vi "LEDs.vi"(11 "Enum":T1(ring)) -> ()   [LabVIEW 2017]
uses:
  <vilib>/myRIO/Instrument Drivers/Onboard IO/DIO/typedefs/DIO Reference.ctl
  <vilib>/myRIO/Common/Instrument Driver Framework/Utilities/typedefs/myRIO Generic Hardware Reference.ctl
  <vilib>/myRIO/Common/Instrument Driver Framework/Utilities/typedefs/Hardware Version Enum.ctl
  <vilib>/myRIO/Common/Instrument Driver Framework/Utilities/typedefs/myRIO v1.0 Reference.ctl
  <vilib>/myRIO/Common/Instrument Driver Framework/Utilities/typedefs/Generic FPGA Reference.ctl
  <vilib>/myRIO/Common/Instrument Driver Framework/myRIO v1.0/DIO/typedefs/DIO Channels List.ctl
  <vilib>/myRIO/Common/Instrument Driver Framework/myRIO v1.0/DIO/typedefs/DIO Channels Enum.ctl
  <vilib>/userdefined/High Color/nirio_resource_hc.ctl
  <vilib>/myRIO/Common/Instrument Driver Framework/Utilities/vis/Is FPGA Ref Available.vi
  <vilib>/myRIO/Common/Instrument Driver Framework/myRIO v1.0/DIO/vis/myRIO v1.1 Open DIO.vi
  <vilib>/myRIO/Instrument Drivers/Onboard IO/DIO/vis/Write.vi
  <vilib>/myRIO/Common/Instrument Driver Framework/Utilities/vis/Validate Channels.vi
  <vilib>/myRIO/Common/Instrument Driver Framework/myRIO v1.0/DIO/vis/myRIO v1.0 Reserve DIO.vi
  <vilib>/myRIO/Common/Instrument Driver Framework/myRIO v1.0/Resource Manager/vis/myRIO v1.0 Reserve Channel List.vi
  <vilib>/myRIO/Common/Instrument Driver Framework/myRIO v1.0/DIO/vis/myRIO v1.0 Build MUX Configuration DIO.vi
  <vilib>/myRIO/Common/Instrument Driver Framework/myRIO v1.0/Resource Manager/vis/myRIO v1.0 Reserve Channel.vi
  <vilib>/myRIO/Common/Instrument Driver Framework/myRIO v1.0/Resource Manager/vis/myRIO v1.0 Unreserve Channel.vi
  <vilib>/myRIO/Common/Instrument Driver Framework/myRIO v1.0/Resource Manager/vis/myRIO v1.0 Create Configuration List.vi
  <vilib>/myRIO/Common/Instrument Driver Framework/myRIO v1.0/Resource Manager/vis/myRIO v1.0 Build Mutex Name.vi
  <vilib>/Utility/VariantDataType/GetNumericInfo.vi
  <vilib>/Utility/error.llb/Error Cluster From Error Code.vi
  <vilib>/myRIO/Common/Instrument Driver Framework/myRIO v1.0/myRIO v1.1 Open.vi
  <vilib>/myRIO/Common/Instrument Driver Framework/Utilities/vis/IO Manager.vi
  <vilib>/myRIO/Common/Instrument Driver Framework/Utilities/vis/Configuration Manager.vi
  <vilib>/myRIO/Common/Instrument Driver Framework/myRIO v1.0/Resource Manager/vis/myRIO v1.0 Configure IO.vi
  <vilib>/myRIO/Common/Instrument Driver Framework/myRIO v1.0/myRIO v1.0 Close.vi
  <vilib>/myRIO/Common/Instrument Driver Framework/myRIO v1.0/DIO/vis/myRIO v1.0 Write DIO.vi
  <vilib>/myRIO/Express VI/Onboard IO/DO/DO Express VI.xnode
  <vilib>/myRIO/Instrument Drivers/Onboard IO/DIO/vis/myRIO DIO Open.xnode
  <vilib>/myRIO/Instrument Drivers/Onboard IO/DIO/DIO.lvlib
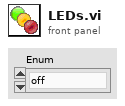
[diagram p1: front panel]
types:
  T1 = enum16{"off", "flash", "top", "middle", "bottom"}
  T2 = typedef "DIO.lvlib/DIO Reference.ctl" = cluster{"myRIO Reference":T3, "DIO Channels List":T7}
  T3 = typedef "myRIO Generic Hardware Reference.ctl" = cluster{"myRIO Model":T4, "myRIO Hardware Reference":T5}
  T4 = typedef "Hardware Version Enum.ctl" = enum16{"Unknown", "myRIO-1900", "myRIO-1950", "roboRIO", "NI ELVIS RIO CM"}
  T5 = typedef "myRIO v1.0 Reference.ctl" = cluster{"Generic FPGA Reference":T6, "Allow multiple opens":bool}
  T6 = typedef "Generic FPGA Reference.ctl" = refnum<k20>
  T7 = typedef "DIO Channels List.ctl" = T8[]
  T8 = typedef "DIO Channels Enum.ctl" = enum16{"Not Connected", "C/DIO0", "C/DIO1", "C/DIO2", "C/DIO3", "C/DIO4", "C/DIO5", "C/DIO6", "C/DIO7", "A/DIO0", "A/DIO1", "A/DIO2", "A/DIO3", "A/DIO4", "A/DIO5", "A/DIO6", "A/DIO7", "A/DIO8", "A/DIO9", "A/DIO10", "A/DIO11", "A/DIO12", "A/DIO13", "A/DIO14", "A/DIO15", "B/DIO0", "B/DIO1", "B/DIO2", "B/DIO3", "B/DIO4", "B/DIO5", "B/DIO6", "B/DIO7", "B/DIO8", "B/DIO9", "B/DIO10", "B/DIO11", "B/DIO12", "B/DIO13", "B/DIO14", "B/DIO15", "LED0", "LED1", "LED2", "LED3", "Button0", "DIO/DIO0", "DIO/DIO1", "DIO/DIO2", "DIO/DIO3", "DIO/DIO4", "DIO/DIO5", "DIO/DIO6", "DIO/DIO7", "DIO/DIO8", "DIO/DIO9", "SPI/CS0", "SPI/CS1", "SPI/CS2", "SPI/CS3", "LED RADIO (Green)", "LED RADIO (Red)", "LED COMM (Green)", "LED COMM (Red)", "LED MODE (Green)", "LED MODE (Red)"}
  T9 = typedef "nirio_resource_hc.ctl" = tag
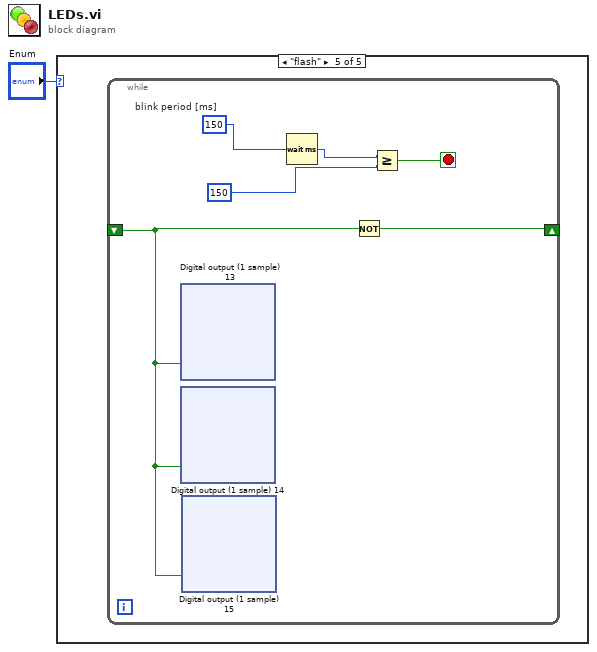
[diagram p0: block diagram]
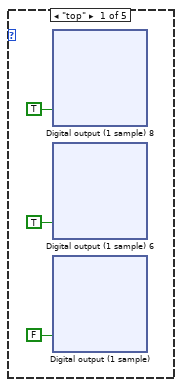
[diagram p2: hidden frame]
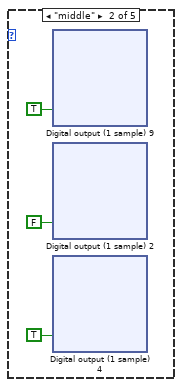
[diagram p3: hidden frame]
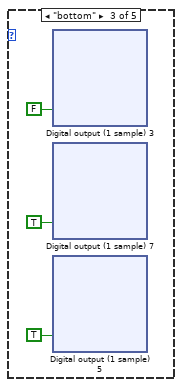
[diagram p4: hidden frame]
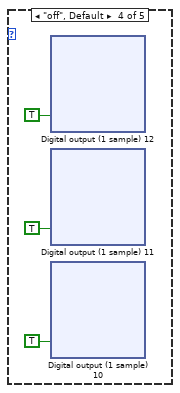
[diagram p5: hidden frame]
diagram:
  n1 = case shown="\"flash\"" "Enum" {
    frame "top" {
      n2 = xnode "Digital output (1 sample) 8"("RED (B/DIO2 (Pin 15))"=TRUE ("RED (A/DIO2 (Pin 15))")) -> ()  [unwired: 1 in, 1 out]
      n3 = xnode "Digital output (1 sample) 6"("YELLOW (B/DIO1 (Pin 13))"=TRUE ("YELLOW (A/DIO1 (Pin 13))")) -> ()  [unwired: 1 in, 1 out]
      n4 = xnode "Digital output (1 sample)"("GREEN (B/DIO0 (Pin 11))"=FALSE ("GREEN (A/DIO0 (Pin 11))")) -> ()  [unwired: 1 in, 1 out]
    }
    frame "middle" {
      n5 = xnode "Digital output (1 sample) 9"("RED (B/DIO2 (Pin 15))"=TRUE ("RED (A/DIO2 (Pin 15))")) -> ()  [unwired: 1 in, 1 out]
      n6 = xnode "Digital output (1 sample) 2"("YELLOW (B/DIO1 (Pin 13))"=FALSE ("YELLOW (A/DIO1 (Pin 13))")) -> ()  [unwired: 1 in, 1 out]
      n7 = xnode "Digital output (1 sample) 4"("GREEN (B/DIO0 (Pin 11))"=TRUE ("GREEN (A/DIO0 (Pin 11))")) -> ()  [unwired: 1 in, 1 out]
    }
    frame "bottom" {
      n8 = xnode "Digital output (1 sample) 3"("RED (B/DIO2 (Pin 15))"=FALSE ("RED (A/DIO2 (Pin 15))")) -> ()  [unwired: 1 in, 1 out]
      n9 = xnode "Digital output (1 sample) 7"("YELLOW (B/DIO1 (Pin 13))"=TRUE ("YELLOW (A/DIO1 (Pin 13))")) -> ()  [unwired: 1 in, 1 out]
      n10 = xnode "Digital output (1 sample) 5"("GREEN (B/DIO0 (Pin 11))"=TRUE ("GREEN (A/DIO0 (Pin 11))")) -> ()  [unwired: 1 in, 1 out]
    }
    frame "off", Default {
      n11 = xnode "Digital output (1 sample) 12"("RED (B/DIO2 (Pin 15))"=TRUE ("RED (A/DIO2 (Pin 15))")) -> ()  [unwired: 1 in, 1 out]
      n12 = xnode "Digital output (1 sample) 11"("YELLOW (B/DIO1 (Pin 13))"=TRUE ("YELLOW (A/DIO1 (Pin 13))")) -> ()  [unwired: 1 in, 1 out]
      n13 = xnode "Digital output (1 sample) 10"("GREEN (B/DIO0 (Pin 11))"=TRUE ("GREEN (A/DIO0 (Pin 11))")) -> ()  [unwired: 1 in, 1 out]
    }
    frame "flash" {
      n14 = while {
        shift-right: [w437] -> _
        shift-left: _ -> [w438]
        stop <- w434 stop-if-true
        w439 = u32 150  # blink period [ms]
        n15 = xnode "Digital output (1 sample) 13"("RED (B/DIO2 (Pin 15))"=w438) -> ()  [unwired: 1 in, 1 out]
        n16 = xnode "Digital output (1 sample) 14"("YELLOW (B/DIO1 (Pin 13))"=w438) -> ()  [unwired: 1 in, 1 out]
        n17 = xnode "Digital output (1 sample) 15"("GREEN (B/DIO0 (Pin 11))"=w438) -> ()  [unwired: 1 in, 1 out]
        n18 = Wait (ms)(milliseconds to wait=w439) -> (millisecond timer value=w436:u32)
        n19 = Not(x=w438) -> (.not. x?=w437:bool)
        n20 = Greater Or Equal?(x=w436, y=u32 150) -> (x >= y?=w434:bool)
      }
    }
  }
